vi "Field vs Slow IV.vi"() -> ()   [LabVIEW 2020]
uses:
  <vilib>/Utility/file.llb/Write Delimited Spreadsheet (DBL).vi
panel:
  in  "Tab Control 2":enum32{"Plot 0", "Plot 1", "Plot 2", "Plot 3"}(tab)
  out "I vs Chan 0":cluster{"Y":dbl[], "Y":dbl[]}[](graph)=[{"Y"=[1.5, 1.505, 1.51, 1.515, 1.52, 1.525, 1.53, 1.535, 1.54, 1.545, 1.55, 1.555, 1.56, 1.565, 1.57, 1.575, 1.58, 1.585, 1.59, 1.595, 1.6, 1.605, 1.61, 1.615, 1.62, 1.625, 1.63, 1.635, 1.6400000000000001, 1.645, 1.65, 1.655, 1.66, 1.665, 1.67, 1.675, 1.68, 1.685, 1.69, 1.695, 1.7, 1.705, 1.71, 1.715, 1.72, 1.725, 1.73, 1.735, 1.74, 1.745, 1.75, 1.755, 1.76, 1.7650000000000001, 1.77, 1.775, 1.78, 1.7850000000000001, 1.79, 1.795, 1.8, 1.805, 1.81, 1.815, 1.82, 1.825, 1.83, 1.835, 1.84, 1.845, 1.85, 1.855, 1.8599999999999999, 1.865, 1.87, 1.875, 1.88, 1.885, 1.8900000000000001, 1.895, 1.9, 1.905, 1.9100000000000001, 1.915, 1.92, 1.925, 1.93, 1.935, 1.94, 1.945, 1.95, 1.955, 1.96, 1.965, 1.97, 1.975, 1.98, 1.9849999999999999, 1.99, 1.995, 2.0, 2.005, 2.01, 2.015, 2.02, 2.025, 2.0300000000000002, 2.035, 2.04, 2.045, 2.05, 2.055, 2.06, 2.065, 2.0700000000000003, 2.075, 2.08, 2.085, 2.09, 2.0949999999999998, 2.1, 2.105, 2.11, 2.115, 2.12, 2.125, 2.13, 2.135, 2.14, 2.145, 2.15, 2.1550000000000002, 2.16, 2.165, 2.17, 2.175, 2.18, 2.185, 2.19, 2.1950000000000003, 2.2, 2.205, 2.21, 2.215, 2.2199999999999998, 2.225, 2.23, 2.235, 2.24, 2.245, 2.25, 2.255, 2.26, 2.265, 2.27, 2.275, 2.2800000000000002, 2.285, 2.29, 2.295, 2.3, 2.305, 2.31, 2.315, 2.3200000000000003, 2.325, 2.33, 2.335, 2.34, 2.3449999999999998, 2.35, 2.355, 2.36, 2.365, 2.37, 2.375, 2.38, 2.385, 2.39, 2.395, 2.4, 2.4050000000000002, 2.41, 2.415, 2.42, 2.425, 2.43, 2.435, 2.44, 2.4450000000000003, 2.45, 2.455, 2.46, 2.465, 2.4699999999999998, 2.475, 2.48, 2.485, 2.49, 2.495, 2.5, 2.505, 2.51, 2.515, 2.52, 2.525, 2.5300000000000002, 2.535, 2.54, 2.545, 2.55, 2.5549999999999997, 2.56, 2.565, 2.5700000000000003, 2.575, 2.58, 2.585, 2.59, 2.5949999999999998, 2.6, 2.605, 2.6100000000000003, 2.615, 2.62, 2.625, 2.63, 2.635, 2.64, 2.645, 2.6500000000000004, 2.6550000000000002, 2.66, 2.665, 2.67, 2.675, 2.6799999999999997, 2.685, 2.69, 2.6950000000000003, 2.7, 2.705, 2.71, 2.715, 2.7199999999999998, 2.725, 2.73, 2.7350000000000003, 2.74, 2.745, 2.75, 2.755, 2.76, 2.765, 2.77, 2.7750000000000004, 2.7800000000000002, 2.785, 2.79, 2.795, 2.8, 2.8049999999999997, 2.81, 2.815, 2.8200000000000003, 2.825, 2.83, 2.835, 2.84, 2.8449999999999998, 2.85, 2.855, 2.8600000000000003, 2.865, 2.87, 2.875, 2.88, 2.885, 2.89, 2.895, 2.9000000000000004, 2.9050000000000002, 2.91, 2.915, 2.92, 2.925, 2.9299999999999997, 2.935, 2.94, 2.9450000000000003, 2.95, 2.955, 2.96, 2.965, 2.9699999999999998, 2.975, 2.98, 2.9850000000000003, 2.99, 2.995, 3.0], "Y"=[6.6156494140625e-06, 6.5995361328125006e-06, 6.860595703125e-06, 6.815966796875001e-06, 6.629296875e-06, 6.725463867187501e-06, 6.89208984375e-06, 6.7604248046875e-06, 6.703466796875001e-06, 6.905004882812501e-06, 7.143994140625e-06, 6.781860351562501e-06, 6.9577392578125e-06, 6.8951171875e-06, 7.09951171875e-06, 7.2299072265625e-06, 7.1348144531250006e-06, 7.0348876953125e-06, 7.0186279296875e-06, 6.8879638671874995e-06, 6.9955078125e-06, 7.0866455078125e-06, 7.0669433593750004e-06, 6.9783691406250005e-06, 6.9769287109375e-06, 7.027465820312501e-06, 7.299096679687501e-06, 7.0621826171875e-06, 7.042236328125e-06, 7.05390625e-06, 7.270654296875e-06, 7.450976562500001e-06, 7.242333984375001e-06, 7.214819335937501e-06, 7.214331054687501e-06, 7.0223388671875e-06, 7.086694335937501e-06, 7.0981201171875e-06, 7.3460693359374996e-06, 7.3974609375e-06, 7.264575195312501e-06, 7.3940673828125e-06, 7.2310302734375e-06, 7.469677734375001e-06, 7.527587890625e-06, 7.409790039062501e-06, 7.722314453125e-06, 7.741162109375e-06, 7.538671875e-06, 7.698876953125e-06, 7.79365234375e-06, 7.7605224609375e-06, 7.908154296875001e-06, 7.778735351562502e-06, 7.8468994140625e-06, 7.7814697265625e-06, 7.9154541015625e-06, 7.78876953125e-06, 7.9025390625e-06, 7.7102783203125e-06, 8.0254638671875e-06, 7.81650390625e-06, 7.7733642578125e-06, 7.838427734375e-06, 8.000756835937501e-06, 7.803369140625e-06, 8.1470947265625e-06, 8.122363281250001e-06, 8.015576171875e-06, 8.0428955078125e-06, 7.7995849609375e-06, 8.1434326171875e-06, 8.0010986328125e-06, 7.897656250000001e-06, 7.827612304687501e-06, 7.766748046874999e-06, 7.85146484375e-06, 7.889453125e-06, 7.968872070312499e-06, 8.0005615234375e-06, 8.2376220703125e-06, 8.1786376953125e-06, 8.2513916015625e-06, 8.29208984375e-06, 8.2388671875e-06, 8.19931640625e-06, 8.2802001953125e-06, 8.443017578125001e-06, 8.449755859375e-06, 8.4138916015625e-06, 8.564306640625e-06, 8.4105224609375e-06, 8.2320068359375e-06, 8.366552734375001e-06, 8.518701171875e-06, 8.652294921875002e-06, 8.6939453125e-06, 8.80498046875e-06, 9.227978515625e-06, 9.0858154296875e-06, 9.2788818359375e-06, 9.3503662109375e-06, 9.485009765625e-06, 9.285717773437502e-06, 9.345336914062502e-06, 9.7904296875e-06, 9.7592041015625e-06, 9.6569580078125e-06, 1.01966552734375e-05, 1.03768798828125e-05, 1.013955078125e-05, 1.0394140625000001e-05, 1.0579418945312501e-05, 1.076220703125e-05, 1.073232421875e-05, 1.1024340820312502e-05, 1.1164453125e-05, 1.1322949218750001e-05, 1.1622363281250002e-05, 1.1904931640625e-05, 1.1911572265625002e-05, 1.2339184570312501e-05, 1.2500537109375002e-05, 1.2740844726562501e-05, 1.285322265625e-05, 1.2884936523437502e-05, 1.3046142578125001e-05, 1.3866577148437502e-05, 1.3682031250000003e-05, 1.4437817382812503e-05, 1.4402294921875001e-05, 1.53095947265625e-05, 1.52098876953125e-05, 1.59145263671875e-05, 1.6001611328125e-05, 1.7141601562500003e-05, 1.7263891601562502e-05, 1.71541259765625e-05, 1.8259204101562504e-05, 1.85321044921875e-05, 1.86347412109375e-05, 1.91985107421875e-05, 1.98390380859375e-05, 2.04806396484375e-05, 2.09681640625e-05, 2.2006640625000004e-05, 2.25154296875e-05, 2.27582275390625e-05, 2.3800146484375003e-05, 2.4407739257812502e-05, 2.4760278320312503e-05, 2.57430419921875e-05, 2.6609887695312503e-05, 2.73911376953125e-05, 2.7119091796875e-05, 2.8339111328125e-05, 2.9722607421875003e-05, 3.0245361328125e-05, 3.0236254882812505e-05, 3.1754150390625003e-05, 3.25618408203125e-05, 3.31111572265625e-05, 3.3728198242187504e-05, 3.4521362304687496e-05, 3.520185546875e-05, 3.54622314453125e-05, 3.66463134765625e-05, 3.7109130859375e-05, 3.7485302734375e-05, 3.8547509765625e-05, 3.904365234375e-05, 3.9046875e-05, 3.998369140625e-05, 4.0939404296875e-05, 4.143056640625e-05, 4.179628906250001e-05, 4.2369970703125e-05, 4.26028564453125e-05, 4.3127124023437505e-05, 4.3738183593750005e-05, 4.3873779296875e-05, 4.4547656250000006e-05, 4.45670166015625e-05, 4.54891357421875e-05, 4.6177490234375e-05, 4.6060302734375006e-05, 4.633154296875e-05, 4.6707592773437505e-05, 4.72677978515625e-05, 4.7176904296875e-05, 4.7945458984375005e-05, 4.8335034179687506e-05, 4.86605224609375e-05, 4.8674536132812504e-05, 4.89802978515625e-05, 4.92022705078125e-05, 4.945415039062501e-05, 4.97037353515625e-05, 5.0124487304687504e-05, 5.0323120117187504e-05, 5.0515185546875e-05, 5.0892187499999996e-05, 5.1154541015625e-05, 5.1278369140625e-05, 5.1231542968750003e-05, 5.130100097656251e-05, 5.158137207031251e-05, 5.185832519531251e-05, 5.20868408203125e-05, 5.22366455078125e-05, 5.2339013671875e-05, 5.23698486328125e-05, 5.247021484375e-05, 5.25740966796875e-05, 5.2685058593750004e-05, 5.271892089843751e-05, 5.29219970703125e-05, 5.2985571289062506e-05, 5.3151660156250005e-05, 5.3482714843750004e-05, 5.3514526367187504e-05, 5.373547363281251e-05, 5.39629638671875e-05, 5.41296142578125e-05, 5.41982177734375e-05, 5.42727783203125e-05, 5.43212646484375e-05, 5.462431640625e-05, 5.489465332031251e-05, 5.47357177734375e-05, 5.5075097656250007e-05, 5.5207519531250006e-05, 5.52376708984375e-05, 5.52714599609375e-05, 5.532636718750001e-05, 5.5555004882812503e-05, 5.55648193359375e-05, 5.558767089843751e-05, 5.5666796875000006e-05, 5.5912084960937505e-05, 5.5835253906250005e-05, 5.6077539062500006e-05, 5.6019506835937504e-05, 5.60676513671875e-05, 5.6107861328125e-05, 5.6332250976562506e-05, 5.65072265625e-05, 5.6557568359375e-05, 5.68264404296875e-05, 5.6969409179687504e-05, 5.6886669921875004e-05, 5.7010302734375e-05, 5.707399902343751e-05, 5.70142822265625e-05, 5.7089843750000005e-05, 5.7226318359375e-05, 5.734260253906251e-05, 5.761708984375001e-05, 5.766303710937501e-05, 5.7710791015625e-05, 5.79302734375e-05, 5.7697778320312504e-05, 5.7987426757812505e-05, 5.823701171875e-05, 5.8305810546875005e-05, 5.8348388671874996e-05, 5.84409912109375e-05, 5.8777392578125e-05, 5.8781958007812496e-05, 5.89344482421875e-05, 5.8952099609375e-05, 5.918017578125e-05, 5.92188720703125e-05, 5.954309082031251e-05, 5.977561035156251e-05, 5.9646166992187505e-05, 5.9729345703125005e-05, 5.9951953125e-05, 5.9855004882812506e-05, 5.9770996093749996e-05, 5.99681640625e-05, 6.007705078125e-05, 6.047041015625e-05, 6.06973388671875e-05, 6.0576123046875e-05, 6.0678247070312496e-05, 6.0798999023437506e-05, 6.08008056640625e-05, 6.0889208984375004e-05, 6.09180908203125e-05, 6.10606201171875e-05, 6.12299560546875e-05, 6.111984863281251e-05, 6.12911376953125e-05, 6.16568603515625e-05, 6.173347167968751e-05, 6.18294921875e-05, 6.208735351562501e-05, 6.21252685546875e-05, 6.212973632812499e-05, 6.2308544921875e-05]}]
  out "Name 0":string="DC Voltage V"
  out "I vs Chan 1":cluster{"Y":dbl[], "Y":dbl[]}[](graph)=[{"Y"=[1.5, 1.505, 1.51, 1.515, 1.52, 1.525, 1.53, 1.535, 1.54, 1.545, 1.55, 1.555, 1.56, 1.565, 1.57, 1.575, 1.58, 1.585, 1.59, 1.595, 1.6, 1.605, 1.61, 1.615, 1.62, 1.625, 1.63, 1.635, 1.6400000000000001, 1.645, 1.65, 1.655, 1.66, 1.665, 1.67, 1.675, 1.68, 1.685, 1.69, 1.695, 1.7, 1.705, 1.71, 1.715, 1.72, 1.725, 1.73, 1.735, 1.74, 1.745, 1.75, 1.755, 1.76, 1.7650000000000001, 1.77, 1.775, 1.78, 1.7850000000000001, 1.79, 1.795, 1.8, 1.805, 1.81, 1.815, 1.82, 1.825, 1.83, 1.835, 1.84, 1.845, 1.85, 1.855, 1.8599999999999999, 1.865, 1.87, 1.875, 1.88, 1.885, 1.8900000000000001, 1.895, 1.9, 1.905, 1.9100000000000001, 1.915, 1.92, 1.925, 1.93, 1.935, 1.94, 1.945, 1.95, 1.955, 1.96, 1.965, 1.97, 1.975, 1.98, 1.9849999999999999, 1.99, 1.995, 2.0, 2.005, 2.01, 2.015, 2.02, 2.025, 2.0300000000000002, 2.035, 2.04, 2.045, 2.05, 2.055, 2.06, 2.065, 2.0700000000000003, 2.075, 2.08, 2.085, 2.09, 2.0949999999999998, 2.1, 2.105, 2.11, 2.115, 2.12, 2.125, 2.13, 2.135, 2.14, 2.145, 2.15, 2.1550000000000002, 2.16, 2.165, 2.17, 2.175, 2.18, 2.185, 2.19, 2.1950000000000003, 2.2, 2.205, 2.21, 2.215, 2.2199999999999998, 2.225, 2.23, 2.235, 2.24, 2.245, 2.25, 2.255, 2.26, 2.265, 2.27, 2.275, 2.2800000000000002, 2.285, 2.29, 2.295, 2.3, 2.305, 2.31, 2.315, 2.3200000000000003, 2.325, 2.33, 2.335, 2.34, 2.3449999999999998, 2.35, 2.355, 2.36, 2.365, 2.37, 2.375, 2.38, 2.385, 2.39, 2.395, 2.4, 2.4050000000000002, 2.41, 2.415, 2.42, 2.425, 2.43, 2.435, 2.44, 2.4450000000000003, 2.45, 2.455, 2.46, 2.465, 2.4699999999999998, 2.475, 2.48, 2.485, 2.49, 2.495, 2.5, 2.505, 2.51, 2.515, 2.52, 2.525, 2.5300000000000002, 2.535, 2.54, 2.545, 2.55, 2.5549999999999997, 2.56, 2.565, 2.5700000000000003, 2.575, 2.58, 2.585, 2.59, 2.5949999999999998, 2.6, 2.605, 2.6100000000000003, 2.615, 2.62, 2.625, 2.63, 2.635, 2.64, 2.645, 2.6500000000000004, 2.6550000000000002, 2.66, 2.665, 2.67, 2.675, 2.6799999999999997, 2.685, 2.69, 2.6950000000000003, 2.7, 2.705, 2.71, 2.715, 2.7199999999999998, 2.725, 2.73, 2.7350000000000003, 2.74, 2.745, 2.75, 2.755, 2.76, 2.765, 2.77, 2.7750000000000004, 2.7800000000000002, 2.785, 2.79, 2.795, 2.8, 2.8049999999999997, 2.81, 2.815, 2.8200000000000003, 2.825, 2.83, 2.835, 2.84, 2.8449999999999998, 2.85, 2.855, 2.8600000000000003, 2.865, 2.87, 2.875, 2.88, 2.885, 2.89, 2.895, 2.9000000000000004, 2.9050000000000002, 2.91, 2.915, 2.92, 2.925, 2.9299999999999997, 2.935, 2.94, 2.9450000000000003, 2.95, 2.955, 2.96, 2.965, 2.9699999999999998, 2.975, 2.98, 2.9850000000000003, 2.99, 2.995, 3.0], "Y"=[1.481296142578125, 1.485899658203125, 1.491623779296875, 1.496372802734375, 1.500607421875, 1.506201171875, 1.512212158203125, 1.516510009765625, 1.520935546875, 1.52574560546875, 1.532031982421875, 1.53548974609375, 1.540796630859375, 1.54504443359375, 1.550413818359375, 1.555810546875, 1.5604111328125, 1.56513671875, 1.570776611328125, 1.575748779296875, 1.579657470703125, 1.586687255859375, 1.590750732421875, 1.596195068359375, 1.6001904296875, 1.60581201171875, 1.610980224609375, 1.614694091796875, 1.6195888671875, 1.624559814453125, 1.63003564453125, 1.635827392578125, 1.639400390625, 1.6446259765625, 1.650548828125, 1.654035400390625, 1.659312255859375, 1.664365478515625, 1.6701484375, 1.674442138671875, 1.67888330078125, 1.68497021484375, 1.689583740234375, 1.69438525390625, 1.69949072265625, 1.7033046875, 1.709611328125, 1.7146865234375, 1.719447021484375, 1.724286376953125, 1.728707763671875, 1.733401123046875, 1.738841796875, 1.744190673828125, 1.749333984375, 1.754213623046875, 1.758762451171875, 1.763666015625, 1.768619873046875, 1.773112060546875, 1.778584228515625, 1.78361376953125, 1.788801513671875, 1.793162353515625, 1.79777880859375, 1.801927490234375, 1.808897216796875, 1.8134384765625, 1.817679931640625, 1.823508544921875, 1.82846533203125, 1.833228271484375, 1.838225341796875, 1.843404296875, 1.848100830078125, 1.852965087890625, 1.858184814453125, 1.862722900390625, 1.868026611328125, 1.873251953125, 1.87840966796875, 1.88210595703125, 1.887539794921875, 1.893552001953125, 1.89667529296875, 1.901953369140625, 1.908353515625, 1.9138330078125, 1.917675048828125, 1.923322998046875, 1.92793505859375, 1.934273681640625, 1.9380302734375, 1.942566162109375, 1.948998779296875, 1.9527333984375, 1.957611572265625, 1.963255126953125, 1.9684384765625, 1.972609130859375, 1.97774560546875, 1.9825537109375, 1.987163818359375, 1.99272412109375, 1.996688232421875, 2.00235546875, 2.007000732421875, 2.011778564453125, 2.016716552734375, 2.0221357421875, 2.026481689453125, 2.031533447265625, 2.03667822265625, 2.041638916015625, 2.046490966796875, 2.051802490234375, 2.056508056640625, 2.061195068359375, 2.066268798828125, 2.071982666015625, 2.0766953125, 2.08216748046875, 2.08670263671875, 2.09073828125, 2.096322265625, 2.1008623046875, 2.106653564453125, 2.112296142578125, 2.116163330078125, 2.120879638671875, 2.126167724609375, 2.131207275390625, 2.1357744140625, 2.141315185546875, 2.146663818359375, 2.151198974609375, 2.1564658203125, 2.16050390625, 2.16619970703125, 2.17108447265625, 2.1764951171875, 2.182198486328125, 2.186181640625, 2.191181884765625, 2.19680859375, 2.201070068359375, 2.206341796875, 2.21065283203125, 2.215697021484375, 2.22130908203125, 2.22514111328125, 2.231263671875, 2.235204833984375, 2.24023681640625, 2.246326416015625, 2.250339599609375, 2.25638818359375, 2.25967626953125, 2.26559912109375, 2.270198974609375, 2.275861328125, 2.28002880859375, 2.28554833984375, 2.289510986328125, 2.294212646484375, 2.29975146484375, 2.304468017578125, 2.309668701171875, 2.314978759765625, 2.31974755859375, 2.324486083984375, 2.328228515625, 2.33425634765625, 2.33995361328125, 2.344055419921875, 2.348734619140625, 2.35476513671875, 2.35883203125, 2.36407421875, 2.369318359375, 2.373428955078125, 2.3782236328125, 2.3842890625, 2.389127685546875, 2.394276123046875, 2.398263427734375, 2.40260302734375, 2.408055908203125, 2.413805908203125, 2.418071533203125, 2.42317724609375, 2.42730517578125, 2.432321533203125, 2.4383212890625, 2.443359375, 2.447465576171875, 2.4527998046875, 2.458234130859375, 2.463433349609375, 2.467795654296875, 2.471888427734375, 2.477741455078125, 2.481700927734375, 2.487224365234375, 2.49161474609375, 2.496494873046875, 2.501940185546875, 2.50732861328125, 2.512439697265625, 2.51685888671875, 2.52212939453125, 2.526584716796875, 2.53218310546875, 2.536430908203125, 2.542002197265625, 2.54634326171875, 2.55148583984375, 2.556789794921875, 2.561865478515625, 2.567234619140625, 2.57208447265625, 2.5763681640625, 2.582333251953125, 2.58724560546875, 2.591645751953125, 2.596749755859375, 2.601959228515625, 2.607040283203125, 2.61256787109375, 2.61584228515625, 2.6220859375, 2.626490478515625, 2.630972900390625, 2.636040771484375, 2.641483154296875, 2.6454052734375, 2.65084765625, 2.655864990234375, 2.660786376953125, 2.6665986328125, 2.671231689453125, 2.6759482421875, 2.6809541015625, 2.6863564453125, 2.691091064453125, 2.69605908203125, 2.70098828125, 2.70492822265625, 2.710500732421875, 2.71611083984375, 2.72056298828125, 2.725668212890625, 2.73026123046875, 2.73534423828125, 2.740166748046875, 2.744230224609375, 2.749697509765625, 2.755395751953125, 2.7598564453125, 2.76503271484375, 2.770073486328125, 2.77452294921875, 2.780376708984375, 2.784783203125, 2.790275146484375, 2.79453515625, 2.7993388671875, 2.80516748046875, 2.8095849609375, 2.814790283203125, 2.8197080078125, 2.8248427734375, 2.8291279296875, 2.833797607421875, 2.840931884765625, 2.84431787109375, 2.84849755859375, 2.855468017578125, 2.85949609375, 2.864020751953125, 2.8692666015625, 2.874175537109375, 2.879315673828125, 2.88516943359375, 2.8895234375, 2.89448828125, 2.899353515625, 2.903724853515625, 2.908484619140625, 2.913658203125, 2.919510498046875, 2.9251630859375, 2.92857080078125, 2.934135986328125, 2.939365234375, 2.943295166015625, 2.94798046875, 2.9540498046875, 2.95862841796875, 2.963914794921875, 2.9681767578125]}]
  out "Name 1":string="DC current uA"
  out "I vs Chan 2":cluster{"Y":dbl[], "Y":dbl[]}[](graph)=[{"Y"=[1.5, 1.505, 1.51, 1.515, 1.52, 1.525, 1.53, 1.535, 1.54, 1.545, 1.55, 1.555, 1.56, 1.565, 1.57, 1.575, 1.58, 1.585, 1.59, 1.595, 1.6, 1.605, 1.61, 1.615, 1.62, 1.625, 1.63, 1.635, 1.6400000000000001, 1.645, 1.65, 1.655, 1.66, 1.665, 1.67, 1.675, 1.68, 1.685, 1.69, 1.695, 1.7, 1.705, 1.71, 1.715, 1.72, 1.725, 1.73, 1.735, 1.74, 1.745, 1.75, 1.755, 1.76, 1.7650000000000001, 1.77, 1.775, 1.78, 1.7850000000000001, 1.79, 1.795, 1.8, 1.805, 1.81, 1.815, 1.82, 1.825, 1.83, 1.835, 1.84, 1.845, 1.85, 1.855, 1.8599999999999999, 1.865, 1.87, 1.875, 1.88, 1.885, 1.8900000000000001, 1.895, 1.9, 1.905, 1.9100000000000001, 1.915, 1.92, 1.925, 1.93, 1.935, 1.94, 1.945, 1.95, 1.955, 1.96, 1.965, 1.97, 1.975, 1.98, 1.9849999999999999, 1.99, 1.995, 2.0, 2.005, 2.01, 2.015, 2.02, 2.025, 2.0300000000000002, 2.035, 2.04, 2.045, 2.05, 2.055, 2.06, 2.065, 2.0700000000000003, 2.075, 2.08, 2.085, 2.09, 2.0949999999999998, 2.1, 2.105, 2.11, 2.115, 2.12, 2.125, 2.13, 2.135, 2.14, 2.145, 2.15, 2.1550000000000002, 2.16, 2.165, 2.17, 2.175, 2.18, 2.185, 2.19, 2.1950000000000003, 2.2, 2.205, 2.21, 2.215, 2.2199999999999998, 2.225, 2.23, 2.235, 2.24, 2.245, 2.25, 2.255, 2.26, 2.265, 2.27, 2.275, 2.2800000000000002, 2.285, 2.29, 2.295, 2.3, 2.305, 2.31, 2.315, 2.3200000000000003, 2.325, 2.33, 2.335, 2.34, 2.3449999999999998, 2.35, 2.355, 2.36, 2.365, 2.37, 2.375, 2.38, 2.385, 2.39, 2.395, 2.4, 2.4050000000000002, 2.41, 2.415, 2.42, 2.425, 2.43, 2.435, 2.44, 2.4450000000000003, 2.45, 2.455, 2.46, 2.465, 2.4699999999999998, 2.475, 2.48, 2.485, 2.49, 2.495, 2.5, 2.505, 2.51, 2.515, 2.52, 2.525, 2.5300000000000002, 2.535, 2.54, 2.545, 2.55, 2.5549999999999997, 2.56, 2.565, 2.5700000000000003, 2.575, 2.58, 2.585, 2.59, 2.5949999999999998, 2.6, 2.605, 2.6100000000000003, 2.615, 2.62, 2.625, 2.63, 2.635, 2.64, 2.645, 2.6500000000000004, 2.6550000000000002, 2.66, 2.665, 2.67, 2.675, 2.6799999999999997, 2.685, 2.69, 2.6950000000000003, 2.7, 2.705, 2.71, 2.715, 2.7199999999999998, 2.725, 2.73, 2.7350000000000003, 2.74, 2.745, 2.75, 2.755, 2.76, 2.765, 2.77, 2.7750000000000004, 2.7800000000000002, 2.785, 2.79, 2.795, 2.8, 2.8049999999999997, 2.81, 2.815, 2.8200000000000003, 2.825, 2.83, 2.835, 2.84, 2.8449999999999998, 2.85, 2.855, 2.8600000000000003, 2.865, 2.87, 2.875, 2.88, 2.885, 2.89, 2.895, 2.9000000000000004, 2.9050000000000002, 2.91, 2.915, 2.92, 2.925, 2.9299999999999997, 2.935, 2.94, 2.9450000000000003, 2.95, 2.955, 2.96, 2.965, 2.9699999999999998, 2.975, 2.98, 2.9850000000000003, 2.99, 2.995, 3.0], "Y"=[0.000686767578125, 0.0008046875, 0.00070556640625, 0.000737060546875, 0.0007373046875, 0.00081640625, 0.0007685546875, 0.000751708984375, 0.000693115234375, 0.000705078125, 0.000750732421875, 0.00069140625, 0.000772216796875, 0.000817626953125, 0.000669677734375, 0.00075830078125, 0.00072509765625, 0.000730224609375, 0.000702392578125, 0.000646240234375, 0.0007041015625, 0.000651611328125, 0.000765380859375, 0.0007802734375, 0.000746337890625, 0.000791015625, 0.000671875, 0.000685791015625, 0.000728759765625, 0.0007724609375, 0.00074853515625, 0.00071533203125, 0.000746337890625, 0.000707275390625, 0.0006455078125, 0.000671630859375, 0.000740478515625, 0.00071240234375, 0.000741455078125, 0.000736328125, 0.000663330078125, 0.00077734375, 0.000770263671875, 0.0007431640625, 0.000709716796875, 0.000694580078125, 0.000658203125, 0.000761962890625, 0.000716796875, 0.0007294921875, 0.000708740234375, 0.000719970703125, 0.000759765625, 0.0007119140625, 0.00072509765625, 0.000751220703125, 0.00073046875, 0.00076220703125, 0.000786376953125, 0.000660400390625, 0.00076904296875, 0.0007451171875, 0.000749267578125, 0.000729248046875, 0.000765869140625, 0.00072314453125, 0.00068115234375, 0.0006806640625, 0.00074951171875, 0.000646484375, 0.000708984375, 0.00069287109375, 0.000790283203125, 0.00073828125, 0.00075634765625, 0.0007880859375, 0.00071142578125, 0.00074853515625, 0.000688232421875, 0.00076806640625, 0.000766845703125, 0.000721435546875, 0.00076416015625, 0.000644287109375, 0.0007109375, 0.000718505859375, 0.000741455078125, 0.00070166015625, 0.00070458984375, 0.0007685546875, 0.000790283203125, 0.000731201171875, 0.000719970703125, 0.00076123046875, 0.000741943359375, 0.00072509765625, 0.000703857421875, 0.000728759765625, 0.00071826171875, 0.000761962890625, 0.000738525390625, 0.00075390625, 0.00076953125, 0.000770751953125, 0.000716064453125, 0.000763916015625, 0.000642578125, 0.000780029296875, 0.000813232421875, 0.000796875, 0.0007158203125, 0.0007373046875, 0.000729736328125, 0.00072314453125, 0.000728759765625, 0.000743896484375, 0.0007421875, 0.000664794921875, 0.000705322265625, 0.000717041015625, 0.000751953125, 0.0006923828125, 0.000789794921875, 0.000712890625, 0.000678466796875, 0.00070703125, 0.00078125, 0.000693359375, 0.00076123046875, 0.00076513671875, 0.000746826171875, 0.000696533203125, 0.000743408203125, 0.000717529296875, 0.000701904296875, 0.000748046875, 0.00071044921875, 0.000751708984375, 0.000792724609375, 0.000766357421875, 0.000755859375, 0.00078759765625, 0.000754150390625, 0.00072412109375, 0.000657470703125, 0.0007158203125, 0.000760986328125, 0.00077197265625, 0.000725341796875, 0.000772705078125, 0.0006953125, 0.00079443359375, 0.000690673828125, 0.00071484375, 0.0006767578125, 0.00067626953125, 0.000764892578125, 0.000652099609375, 0.000696533203125, 0.0007265625, 0.000674072265625, 0.000666748046875, 0.0007431640625, 0.00070703125, 0.0007421875, 0.000761962890625, 0.000734619140625, 0.00068212890625, 0.000670166015625, 0.00069287109375, 0.000703125, 0.000656005859375, 0.000713134765625, 0.000716552734375, 0.00072412109375, 0.000741943359375, 0.000707275390625, 0.0007041015625, 0.000737548828125, 0.00070263671875, 0.0007080078125, 0.000760986328125, 0.00073876953125, 0.000724609375, 0.000735595703125, 0.0006669921875, 0.00069287109375, 0.000710693359375, 0.000724365234375, 0.000623779296875, 0.000720458984375, 0.000756591796875, 0.0008076171875, 0.00076123046875, 0.000697509765625, 0.00073974609375, 0.00069873046875, 0.000677001953125, 0.00069970703125, 0.000749755859375, 0.00071435546875, 0.0007197265625, 0.00066015625, 0.000712646484375, 0.000734619140625, 0.00070849609375, 0.00071875, 0.000677490234375, 0.0007197265625, 0.000694091796875, 0.000782958984375, 0.000737060546875, 0.000674560546875, 0.000730712890625, 0.0007265625, 0.000721435546875, 0.000716552734375, 0.00073388671875, 0.00065234375, 0.0007294921875, 0.0007119140625, 0.000756591796875, 0.000716796875, 0.00078857421875, 0.00064599609375, 0.000800537109375, 0.000707275390625, 0.00069189453125, 0.000704345703125, 0.000674560546875, 0.000740234375, 0.0007607421875, 0.000720458984375, 0.000779052734375, 0.0007216796875, 0.0007333984375, 0.000665283203125, 0.000680908203125, 0.000768798828125, 0.00070654296875, 0.000694091796875, 0.00066259765625, 0.000719482421875, 0.000688232421875, 0.000730712890625, 0.0006787109375, 0.000701416015625, 0.00065576171875, 0.000739990234375, 0.00077685546875, 0.00076953125, 0.00064892578125, 0.000725830078125, 0.0006650390625, 0.000781005859375, 0.000702392578125, 0.00065673828125, 0.00071630859375, 0.000720703125, 0.00068115234375, 0.000761474609375, 0.000705078125, 0.00065771484375, 0.000735595703125, 0.000689453125, 0.000717529296875, 0.000713623046875, 0.00070361328125, 0.000772216796875, 0.000658447265625, 0.00068603515625, 0.000721435546875, 0.000724609375, 0.000708740234375, 0.000685546875, 0.00075537109375, 0.00075732421875, 0.000718994140625, 0.0007041015625, 0.0007265625, 0.000692138671875, 0.000771484375, 0.000732177734375, 0.000716064453125, 0.000693603515625, 0.00069091796875, 0.000716552734375, 0.000638427734375, 0.0006689453125, 0.000714111328125, 0.0007451171875, 0.0006875, 0.000751220703125, 0.000694580078125, 0.000660888671875, 0.0006923828125, 0.00068701171875, 0.0006552734375, 0.00069140625, 0.000733154296875, 0.000695068359375]}]
  out "Name 2":string="dV V"
  out "I vs Chan 3":cluster{"Y":dbl[], "Y":dbl[]}[](graph)=[{"Y"=[1.5, 1.505, 1.51, 1.515, 1.52, 1.525, 1.53, 1.535, 1.54, 1.545, 1.55, 1.555, 1.56, 1.565, 1.57, 1.575, 1.58, 1.585, 1.59, 1.595, 1.6, 1.605, 1.61, 1.615, 1.62, 1.625, 1.63, 1.635, 1.6400000000000001, 1.645, 1.65, 1.655, 1.66, 1.665, 1.67, 1.675, 1.68, 1.685, 1.69, 1.695, 1.7, 1.705, 1.71, 1.715, 1.72, 1.725, 1.73, 1.735, 1.74, 1.745, 1.75, 1.755, 1.76, 1.7650000000000001, 1.77, 1.775, 1.78, 1.7850000000000001, 1.79, 1.795, 1.8, 1.805, 1.81, 1.815, 1.82, 1.825, 1.83, 1.835, 1.84, 1.845, 1.85, 1.855, 1.8599999999999999, 1.865, 1.87, 1.875, 1.88, 1.885, 1.8900000000000001, 1.895, 1.9, 1.905, 1.9100000000000001, 1.915, 1.92, 1.925, 1.93, 1.935, 1.94, 1.945, 1.95, 1.955, 1.96, 1.965, 1.97, 1.975, 1.98, 1.9849999999999999, 1.99, 1.995, 2.0, 2.005, 2.01, 2.015, 2.02, 2.025, 2.0300000000000002, 2.035, 2.04, 2.045, 2.05, 2.055, 2.06, 2.065, 2.0700000000000003, 2.075, 2.08, 2.085, 2.09, 2.0949999999999998, 2.1, 2.105, 2.11, 2.115, 2.12, 2.125, 2.13, 2.135, 2.14, 2.145, 2.15, 2.1550000000000002, 2.16, 2.165, 2.17, 2.175, 2.18, 2.185, 2.19, 2.1950000000000003, 2.2, 2.205, 2.21, 2.215, 2.2199999999999998, 2.225, 2.23, 2.235, 2.24, 2.245, 2.25, 2.255, 2.26, 2.265, 2.27, 2.275, 2.2800000000000002, 2.285, 2.29, 2.295, 2.3, 2.305, 2.31, 2.315, 2.3200000000000003, 2.325, 2.33, 2.335, 2.34, 2.3449999999999998, 2.35, 2.355, 2.36, 2.365, 2.37, 2.375, 2.38, 2.385, 2.39, 2.395, 2.4, 2.4050000000000002, 2.41, 2.415, 2.42, 2.425, 2.43, 2.435, 2.44, 2.4450000000000003, 2.45, 2.455, 2.46, 2.465, 2.4699999999999998, 2.475, 2.48, 2.485, 2.49, 2.495, 2.5, 2.505, 2.51, 2.515, 2.52, 2.525, 2.5300000000000002, 2.535, 2.54, 2.545, 2.55, 2.5549999999999997, 2.56, 2.565, 2.5700000000000003, 2.575, 2.58, 2.585, 2.59, 2.5949999999999998, 2.6, 2.605, 2.6100000000000003, 2.615, 2.62, 2.625, 2.63, 2.635, 2.64, 2.645, 2.6500000000000004, 2.6550000000000002, 2.66, 2.665, 2.67, 2.675, 2.6799999999999997, 2.685, 2.69, 2.6950000000000003, 2.7, 2.705, 2.71, 2.715, 2.7199999999999998, 2.725, 2.73, 2.7350000000000003, 2.74, 2.745, 2.75, 2.755, 2.76, 2.765, 2.77, 2.7750000000000004, 2.7800000000000002, 2.785, 2.79, 2.795, 2.8, 2.8049999999999997, 2.81, 2.815, 2.8200000000000003, 2.825, 2.83, 2.835, 2.84, 2.8449999999999998, 2.85, 2.855, 2.8600000000000003, 2.865, 2.87, 2.875, 2.88, 2.885, 2.89, 2.895, 2.9000000000000004, 2.9050000000000002, 2.91, 2.915, 2.92, 2.925, 2.9299999999999997, 2.935, 2.94, 2.9450000000000003, 2.95, 2.955, 2.96, 2.965, 2.9699999999999998, 2.975, 2.98, 2.9850000000000003, 2.99, 2.995, 3.0], "Y"=[0.00172412109375, 0.001721435546875, 0.00168603515625, 0.00166357421875, 0.00168310546875, 0.001632080078125, 0.001675048828125, 0.0017109375, 0.0016943359375, 0.001686767578125, 0.00173095703125, 0.001705322265625, 0.001647705078125, 0.001672607421875, 0.0016767578125, 0.0016572265625, 0.00168896484375, 0.0016826171875, 0.001687255859375, 0.001647705078125, 0.00169775390625, 0.00166357421875, 0.00173388671875, 0.0017080078125, 0.001659912109375, 0.00169140625, 0.0016962890625, 0.001697509765625, 0.001662841796875, 0.00162939453125, 0.0017177734375, 0.001651611328125, 0.00163818359375, 0.001712646484375, 0.001668701171875, 0.00170361328125, 0.001758056640625, 0.001680908203125, 0.001697265625, 0.001639404296875, 0.001704833984375, 0.001695556640625, 0.001661376953125, 0.001728515625, 0.001750244140625, 0.001653564453125, 0.001721435546875, 0.0017109375, 0.001679443359375, 0.001676513671875, 0.0016865234375, 0.001657958984375, 0.001687255859375, 0.001693115234375, 0.00168798828125, 0.00168359375, 0.00169287109375, 0.001712158203125, 0.00172216796875, 0.001672119140625, 0.001680419921875, 0.001711181640625, 0.001709716796875, 0.00168896484375, 0.001654052734375, 0.001686279296875, 0.00166357421875, 0.0016826171875, 0.001654296875, 0.001711181640625, 0.001636474609375, 0.001697509765625, 0.00170361328125, 0.001681884765625, 0.001663818359375, 0.00164111328125, 0.001682373046875, 0.00169189453125, 0.001673095703125, 0.001668701171875, 0.001681884765625, 0.00164404296875, 0.001693115234375, 0.00165283203125, 0.00164501953125, 0.00166064453125, 0.001638427734375, 0.0016728515625, 0.00165087890625, 0.001656005859375, 0.001697265625, 0.001666259765625, 0.001629638671875, 0.001615966796875, 0.00169580078125, 0.00165869140625, 0.001694580078125, 0.0016787109375, 0.001703125, 0.00165966796875, 0.00172705078125, 0.001748779296875, 0.00166015625, 0.00170166015625, 0.0016787109375, 0.001710693359375, 0.00170654296875, 0.001665771484375, 0.00166455078125, 0.001759765625, 0.00169921875, 0.00166162109375, 0.00172705078125, 0.001671875, 0.001734619140625, 0.001705322265625, 0.001665283203125, 0.001691162109375, 0.001689208984375, 0.001666748046875, 0.001759033203125, 0.001675048828125, 0.001667236328125, 0.0016767578125, 0.001724853515625, 0.00165673828125, 0.001669189453125, 0.001679931640625, 0.001667724609375, 0.00168603515625, 0.001764404296875, 0.00171826171875, 0.001695068359375, 0.00172802734375, 0.00165771484375, 0.001701904296875, 0.001660888671875, 0.001697265625, 0.00170556640625, 0.00173388671875, 0.00172314453125, 0.001640380859375, 0.001629638671875, 0.00165966796875, 0.00167529296875, 0.001738525390625, 0.001657958984375, 0.001710693359375, 0.00167724609375, 0.001677490234375, 0.00166943359375, 0.001637939453125, 0.001658935546875, 0.001703125, 0.001694091796875, 0.001676025390625, 0.00168310546875, 0.00167578125, 0.001646240234375, 0.001751953125, 0.0016689453125, 0.00170361328125, 0.001697021484375, 0.001707763671875, 0.001684326171875, 0.001719970703125, 0.001631591796875, 0.001638427734375, 0.001682861328125, 0.00175537109375, 0.0016767578125, 0.0017099609375, 0.001689697265625, 0.00172119140625, 0.001761962890625, 0.001656982421875, 0.001688232421875, 0.001677978515625, 0.00167919921875, 0.0016611328125, 0.001636962890625, 0.001694580078125, 0.001733154296875, 0.001700927734375, 0.001701171875, 0.001706298828125, 0.00170263671875, 0.001689208984375, 0.001663818359375, 0.001662353515625, 0.0017177734375, 0.00167041015625, 0.001654052734375, 0.001680419921875, 0.0017236328125, 0.0016943359375, 0.0016875, 0.001731201171875, 0.001698974609375, 0.001718505859375, 0.001677001953125, 0.001695556640625, 0.001710693359375, 0.001684814453125, 0.001716064453125, 0.001660400390625, 0.001641845703125, 0.001656982421875, 0.001673095703125, 0.001685302734375, 0.00160498046875, 0.00165380859375, 0.0017490234375, 0.001673583984375, 0.001743408203125, 0.00170361328125, 0.001679931640625, 0.001680419921875, 0.001702392578125, 0.001679931640625, 0.001658935546875, 0.001725341796875, 0.001708251953125, 0.001735107421875, 0.001676025390625, 0.001728515625, 0.00171533203125, 0.0016328125, 0.001673583984375, 0.001707275390625, 0.001645751953125, 0.001700927734375, 0.001675537109375, 0.001673583984375, 0.001682861328125, 0.001618408203125, 0.001680908203125, 0.0016806640625, 0.00168115234375, 0.00167041015625, 0.00169873046875, 0.00166552734375, 0.00168701171875, 0.0017099609375, 0.00169921875, 0.001651123046875, 0.001683837890625, 0.0016748046875, 0.001654541015625, 0.001683349609375, 0.001668212890625, 0.00162548828125, 0.00167333984375, 0.0016435546875, 0.0016689453125, 0.0017265625, 0.001734619140625, 0.001675537109375, 0.0016943359375, 0.001693359375, 0.001719970703125, 0.001652099609375, 0.001674560546875, 0.001696533203125, 0.001704345703125, 0.001668212890625, 0.001690185546875, 0.001684326171875, 0.001725830078125, 0.0017099609375, 0.001635009765625, 0.00161328125, 0.001689208984375, 0.00168017578125, 0.001648681640625, 0.0016796875, 0.00165576171875, 0.0016513671875, 0.001722412109375, 0.00173046875, 0.001647216796875, 0.00166748046875, 0.00167236328125, 0.001693603515625, 0.001658447265625, 0.001661865234375, 0.00169970703125, 0.00171142578125, 0.001665771484375, 0.001665771484375, 0.001686279296875, 0.00163916015625, 0.00164208984375, 0.001709228515625, 0.0016494140625, 0.001640869140625, 0.001671142578125, 0.001713134765625, 0.001692626953125, 0.00167919921875, 0.0016806640625]}]
  out "Name 3":string="dI uA"
  in  "Tab Control":T1(tab)=enum."Field"
  in  "cRIO IP":string="//172.22.11.2"
  in  "Reading Average times":i32=1000
  in  "Current Start uA":dbl=1.5
  in  "Current Range uA":dbl=1.5
  in  "Current Step uA":dbl=0.005
  in  "Current output Scale factor":dbl=1.0
  in  "Ramp type":string(combo)="Range"
  in  "Ramp up first T":bool=TRUE
  in  "AO Channel":string(combo)="AO0"
  in  "Delay Time s":dbl=0.15 caption="Delay Time (s)"
  in  "Channel name 0":string(combo)="DC Voltage V"
  in  "Scale factor0":dbl=0.0001
  in  "Chan 1":bool=TRUE
  in  "Channel name 1":string(combo)="DC current uA"
  in  "Scale factor1":dbl=1.0
  in  "Chan 2":bool
  in  "Channel name 2":string(combo)="dV V"
  in  "Scale factor2":dbl=1.0
  in  "Chan 3":bool
  in  "Channel name 3":string(combo)="dI uA"
  in  "Scale factor3":dbl=1.0
  in  "Contour plot folder":path=path "C:/Users/gyue/Desktop/Data folder 20210720"
  in  "Book name":string="book723"
  in  "Current VI path":path=path "C:/Users/gyue/Box/Guang Yue uiuc research box folder/Labview/cRIO related/Field vs Slow IV.vi"
  out "Current Field mT":dbl=0.30000000000000004
  in  "stop":bool
  in  "Ramp up first T 2":bool=TRUE
  in  "Ramp type 2":string(combo)="Range"
  in  "Field Origin mT":dbl=0.2 format="%#_13g"
  in  "Field step mT":dbl=0.0005 format="%#_13g"
  in  "Field Radius mT":dbl=0.1 format="%#_13g"
  in  "Field Rate mT per sec":dbl=0.1 format="%#_13g"
  in  "Magnet Device Select":string(combo)="NI DAQ Controlled V to I source"
  out "error out":errorcluster
  # "Voltage x factor=uA"
  # "Voltage x factor=actual"
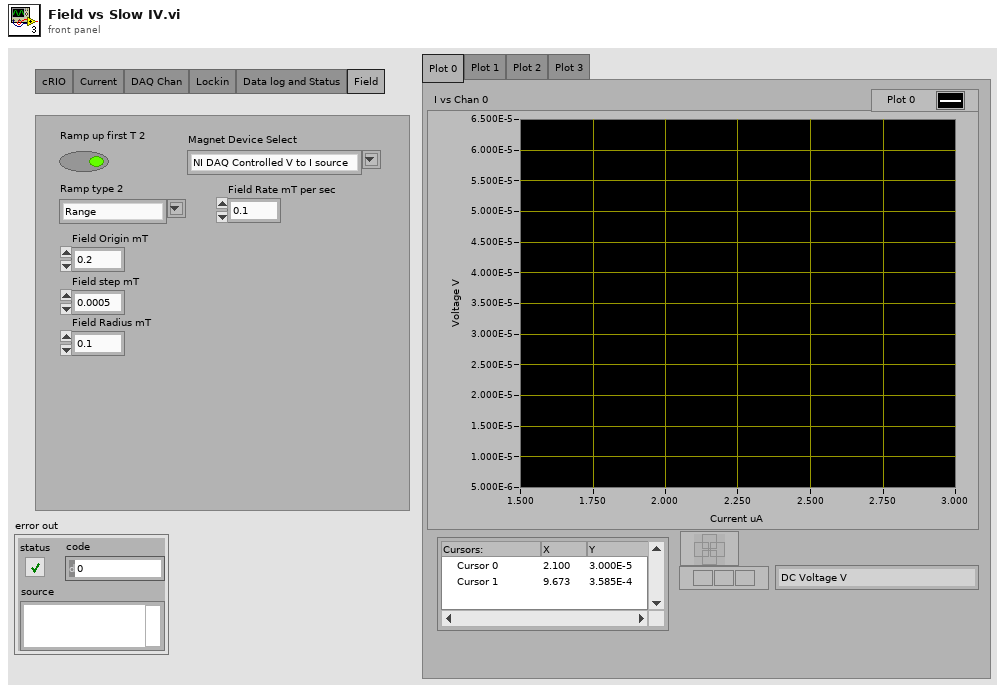
[diagram p1: front panel]
types:
  T1 = enum32{"cRIO", "Current", "DAQ Chan", "Lockin", "Data log and Status", "Field"}
  T2 = cluster{"AI0":dbl, "AI1":dbl, "AI2":dbl, "AI3":dbl}
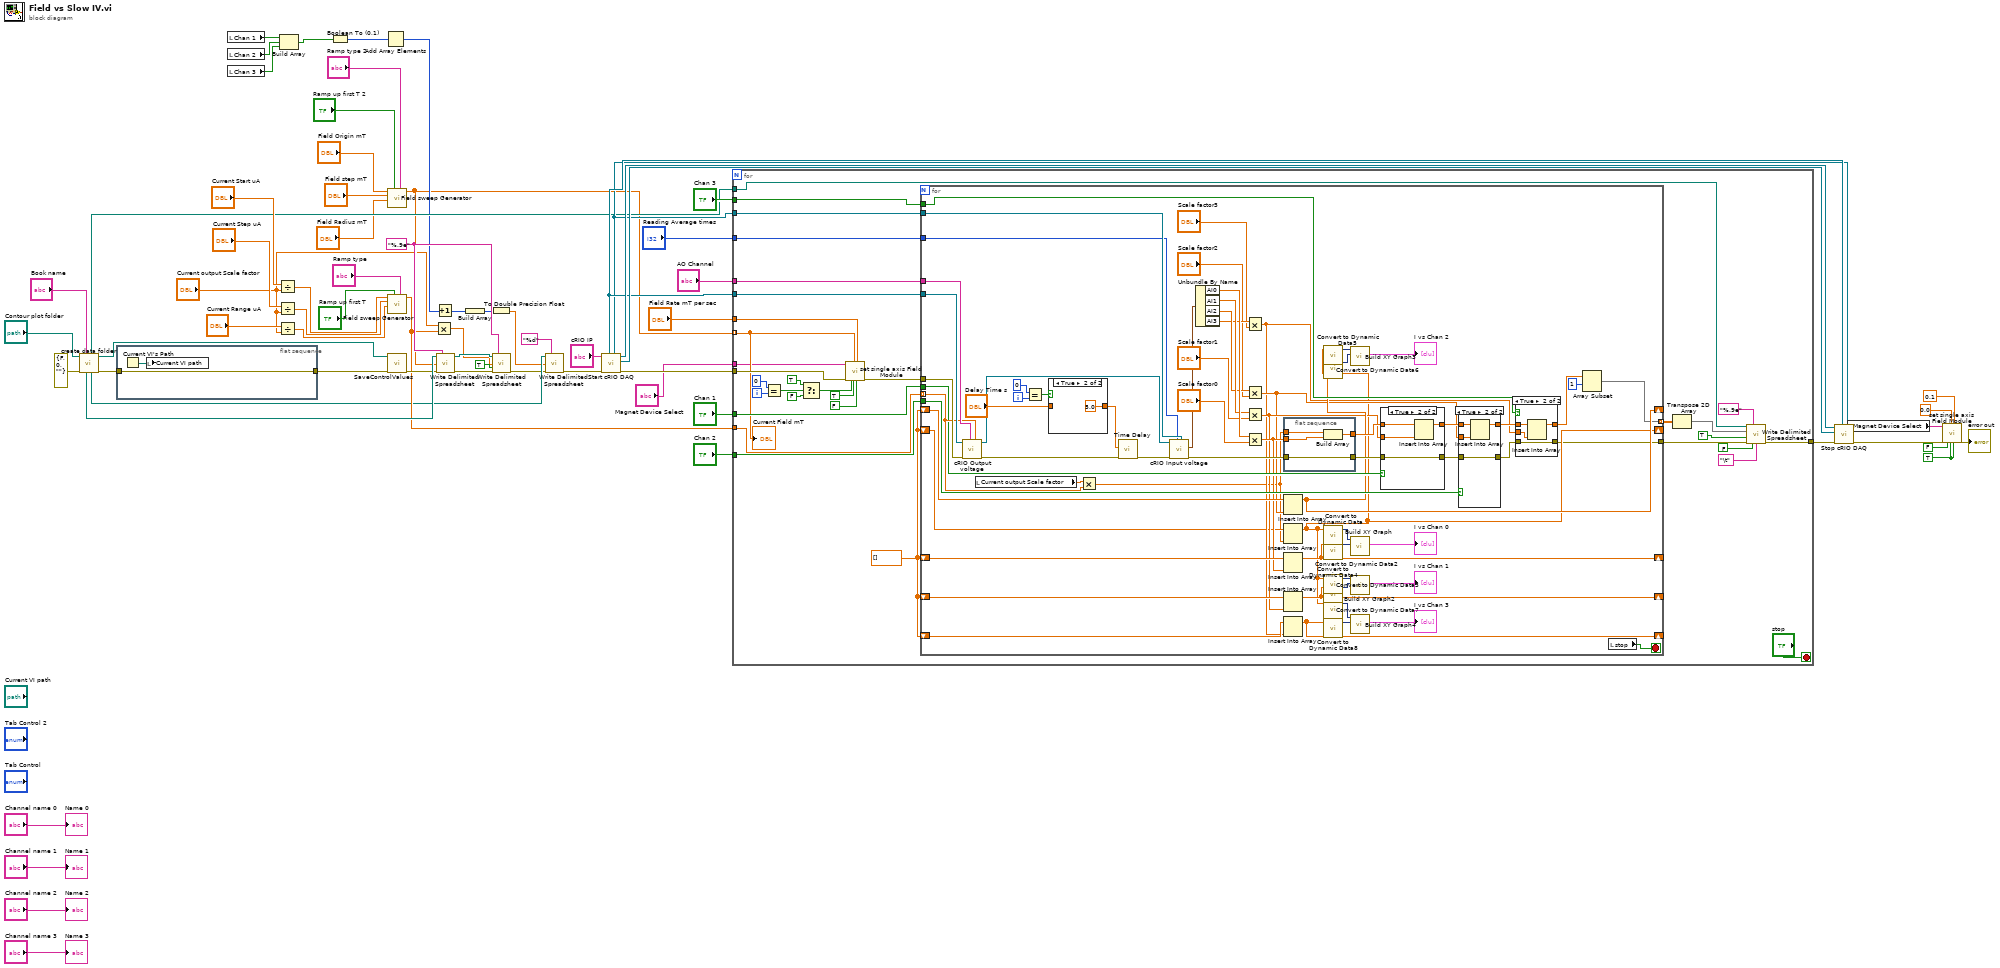
[diagram p0: block diagram]
diagram:
  w2 = TRUE ("final")
  w30 = "%.9e" ("format (%.3f)")
  n1 = call "create data folder.vi"("Name"="Book name", "error in"=errorcluster {"status"=FALSE, "code"=0, "source"=""}, "Contour plot folder"="Contour plot folder") -> ("error out"=w39:errorcluster, "xml path"=w41:path, "book par"=w24:path, "IV path"=w40:path, "Field path"=w37:path)  [unwired: 4 in]
  n2 = flat-sequence {
    tunnel: w39 -> [w69]
    tunnel: [w69] -> w38
    frame #0 {
      n3 = Current VI's Path() -> (path=w70:path)
      n4 = local write "Current VI path"(w70) -> ()
    }
  }
  n5 = local read "Chan 1"() -> (w22:bool)
  n6 = local read "Chan 2"() -> (w21:bool)
  n7 = local read "Chan 3"() -> (w20:bool)
  n8 = Divide(x="Current Start uA", y="Current output Scale factor") -> (x/y=w60:dbl)
  n9 = Divide(x="Current Step uA", y="Current output Scale factor") -> (x/y=w59:dbl)
  n10 = Divide(x="Current Range uA", y="Current output Scale factor") -> (x/y=w58:dbl)
  n11 = Build Array(w22, w21, w20) -> (w19:bool[])
  n12 = Boolean To (0,1)(Boolean=w19) -> (0, 1=w18:i16[])
  n13 = Add Array Elements(numeric array=w18) -> (sum=w17:i16)
  n14 = call "Field sweep Generator.vi"("Ramp type"="Ramp type 2", "Ramp up first T"="Ramp up first T 2", "Field Radius"="Field Radius mT", "Field step"="Field step mT", "Field Origin"="Field Origin mT") -> ("output array"=w12:dbl[])  [unwired: 6 in]
  n15 = call "Field sweep Generator.vi"("Ramp type"="Ramp type", "Ramp up first T"="Ramp up first T", "Field Radius"=w58, "Field step"=w59, "Field Origin"=w60) -> ("output array"=w28:dbl[])  [unwired: 6 in]
  n16 = call "SaveControlValues.vi"("XML File Path"=w41, "error in (no error)"=w38) -> ("error out"=w36:errorcluster)  [unwired: 8 in]
  n17 = Multiply(x="Current output Scale factor", y=w28) -> (x*y=w5:dbl[])
  n18 = Increment(x=w17) -> (x+1=w16:i16)
  n19 = call-poly <vilib>:"Write Delimited Spreadsheet.vi"("file path (dialog if empty)"=w37, "format (%.3f)"=w30, "1D data"=w12, "error in (no error)"=w36) -> ("new file path (Not A Path if cancelled)"=w29:path, "error out"=w26:errorcluster)  [unwired: 10 in]
  n20 = Build Array(w16) -> (w15:i16[])
  n21 = To Double Precision Float(number=w15) -> (double precision float=w14:dbl[])
  n22 = call-poly <vilib>:"Write Delimited Spreadsheet.vi"("file path (dialog if empty)"=w29, "format (%.3f)"=w30, "1D data"=w5, "append to file? (new file:F)"=TRUE, "error in (no error)"=w26) -> ("error out"=w23:errorcluster)  [unwired: 9 in, 1 out]
  n23 = call-poly <vilib>:"Write Delimited Spreadsheet.vi"("file path (dialog if empty)"=w24, "format (%.3f)"="%d", "1D data"=w14, "error in (no error)"=w23) -> ("error out"=w13:errorcluster)  [unwired: 10 in, 1 out]
  n24 = call "Start cRIO DAQ.vi"("error in (no error)"=w13, "cRIO IP"="cRIO IP") -> ("error out"=w57:errorcluster, "vi reference"=w67:refnum<vi>, "application reference"=w68:refnum<vi>, "DAQ_AI_Reader endpoint"=w54:refnum<k21>, "DAQ_CMD_Writer endpoint"=w55:refnum<k21>)  [unwired: 5 in]
  n25 = for {
    tunnel: "AO Channel" -> [w102]
    tunnel: w28 -> [w101]
    tunnel: w55 -> [w100]
    tunnel: w54 -> [w99]
    tunnel: "Chan 1" -> [w98]
    tunnel: "Chan 2" -> [w97]
    tunnel: "Chan 3" -> [w96]
    tunnel: "Reading Average times" -> [w94]
    tunnel: w40 -> [w88]
    tunnel: w12 -> [w90] mode=indexing
    tunnel: w57 -> [w92]
    tunnel: [w82] -> w50
    tunnel: "Field Rate mT per sec" -> [w91]
    tunnel: "Magnet Device Select" -> [w71]
    i -> [w77]
    stop <- "stop" stop-if-true
    w95 = dbl[] []
    n26 = Equal?(x=0, y=w77) -> (x = y?=w75:bool)
    n27 = Select(t=TRUE ("Init"), s=w75, f=FALSE) -> (s? t:f=w72:bool)
    n28 = call "set single axis Field Module.vi"("Magnet Device Select"=w71, "error in (no error)"=w92, "Init"=w72, "Field Target mT"=w90, "Exec"=TRUE, "Field Rate mT per sec"=w91, "final"=FALSE) -> ("error out"=w89:errorcluster)  [unwired: 12 in]
    n29 = for {
      tunnel: w89 -> [w168]
      tunnel: w100 -> [w167]
      tunnel: w102 -> [w166]
      tunnel: w101 -> [w156] mode=indexing
      tunnel: w99 -> [w164]
      tunnel: w98 -> [w147]
      tunnel: w97 -> [w146]
      tunnel: w96 -> [w145]
      shift-right: [w124] -> _
      shift-left: w95 -> [w128]
      shift-right: [w123] -> _
      shift-left: w95 -> [w127]
      shift-right: [w122] -> _
      shift-left: w95 -> [w126]
      shift-right: [w121] -> _
      shift-left: w95 -> [w125]
      shift-right: [w114] -> _
      shift-left: w95 -> [w116]
      tunnel: w94 -> [w113]
      tunnel: [w109] -> w81 mode=indexing
      tunnel: [w112] -> w85
      i -> [w107]
      stop <- w103 stop-if-true
      n30 = call "cRIO Output voltage.vi"("Voltage"=w156, "AO Channel"=w166, "error in (no error)"=w168, "DAQ_CMD_Writer endpoint"=w167) -> ("error out"=w160:errorcluster, "DAQ_CMD_Writer endpoint out"=w165:refnum<k21>)  [unwired: 6 in]
      n31 = local read "Current output Scale factor"() -> (w157:dbl)
      n32 = Equal?(x=0, y=w107) -> (x = y?=w106:bool)
      n33 = case shown="True" w106 {
        tunnel: "Delay Time s" -> [w169 _]
        tunnel: [w169 5.0 ("Delay Time s")] -> w104
        frame False {
        }
        frame True {
        }
      }
      n34 = Multiply(x=w157, y=w156) -> (x*y=w115:dbl)
      n35 = call "Time Delay"("error in (no error)"=w160, "Delay Time (s)"=w104) -> ("error out"=w159:errorcluster)  [unwired: 9 in]
      n36 = call "cRIO Input voltage.vi"("DAQ_AI_Reader endpoint"=w164, "Average"=w113, "error in (no error)"=w159, "DAQ_CMD_Writer endpoint"=w165) -> ("error out"=w142:errorcluster, "output cluster"=w158:T2)  [unwired: 5 in, 1 out]
      n37 = Unbundle By Name(w158) -> ("AI0"=w155:dbl, "AI1"=w154:dbl, "AI2"=w153:dbl, "AI3"=w152:dbl)
      n38 = Multiply(x=w152, y="Scale factor3") -> (x*y=w117:dbl)
      n39 = Multiply(x=w153, y="Scale factor2") -> (x*y=w118:dbl)
      n40 = Multiply(x=w154, y="Scale factor1") -> (x*y=w119:dbl)
      n41 = Multiply(x=w155, y="Scale factor0") -> (x*y=w120:dbl)
      n42 = flat-sequence {
        tunnel: w142 -> [w174]
        tunnel: [w174] -> w141
        tunnel: w120 -> [w172]
        tunnel: [w173] -> w140
        tunnel: w115 -> [w171]
        frame #0 {
          n43 = Build Array(w171, w172) -> (w173:dbl[])
        }
      }
      n44 = Insert Into Array(array=w126, new element=w118) -> (w122:dbl[])  [unwired: 1 in]
      n45 = Insert Into Array(array=w116, new element=w115) -> (w114:dbl[])  [unwired: 1 in]
      n46 = Insert Into Array(array=w128, new element=w120) -> (w124:dbl[])  [unwired: 1 in]
      n47 = Insert Into Array(array=w127, new element=w119) -> (w123:dbl[])  [unwired: 1 in]
      n48 = Insert Into Array(array=w125, new element=w117) -> (w121:dbl[])  [unwired: 1 in]
      n49 = call "Convert to Dynamic Data5"("Array"=w114) -> ("Dynamic Data Type"=w133:dynamicdata)  [unwired: 3 in]
      n50 = call "Convert to Dynamic Data6"("Array"=w122) -> ("Dynamic Data Type"=w134:dynamicdata)  [unwired: 3 in]
      n51 = call "Convert to Dynamic Data"("Array"=w114) -> ("Dynamic Data Type"=w162:dynamicdata)  [unwired: 3 in]
      n52 = call "Convert to Dynamic Data2"("Array"=w124) -> ("Dynamic Data Type"=w163:dynamicdata)  [unwired: 3 in]
      n53 = call "Convert to Dynamic Data3"("Array"=w114) -> ("Dynamic Data Type"=w136:dynamicdata)  [unwired: 3 in]
      n54 = call "Convert to Dynamic Data4"("Array"=w123) -> ("Dynamic Data Type"=w137:dynamicdata)  [unwired: 3 in]
      n55 = call "Convert to Dynamic Data7"("Array"=w114) -> ("Dynamic Data Type"=w130:dynamicdata)  [unwired: 3 in]
      n56 = call "Convert to Dynamic Data8"("Array"=w121) -> ("Dynamic Data Type"=w131:dynamicdata)  [unwired: 3 in]
      n57 = call "Build XY Graph3"("Y Input"=w134, "X Input"=w133) -> ("XY Graph"=→"I vs Chan 2":cluster{"X":dbl[], "Y":dbl[]}[])  [unwired: 8 in, 1 out]
      n58 = call "Build XY Graph"("Y Input"=w163, "X Input"=w162) -> ("XY Graph"=→"I vs Chan 0":cluster{"X":dbl[], "Y":dbl[]}[])  [unwired: 8 in, 1 out]
      n59 = call "Build XY Graph2"("Y Input"=w137, "X Input"=w136) -> ("XY Graph"=→"I vs Chan 1":cluster{"X":dbl[], "Y":dbl[]}[])  [unwired: 8 in, 1 out]
      n60 = call "Build XY Graph4"("Y Input"=w131, "X Input"=w130) -> ("XY Graph"=→"I vs Chan 3":cluster{"X":dbl[], "Y":dbl[]}[])  [unwired: 8 in, 1 out]
      n61 = case shown="True" w147 {
        tunnel: w141 -> [w187 w192]
        tunnel: [w187 w192] -> w144
        tunnel: w140 -> [w188 w191]
        tunnel: w119 -> [_ w190]
        tunnel: [w188 w189] -> w139
        frame False {
        }
        frame True {
          n62 = Insert Into Array(array=w191, new element=w190) -> (w189:dbl[])  [unwired: 1 in]
        }
      }
      n63 = case shown="True" w146 {
        tunnel: w144 -> [w181 w186]
        tunnel: [w181 w186] -> w143
        tunnel: w139 -> [w182 w185]
        tunnel: w118 -> [_ w184]
        tunnel: [w182 w183] -> w138
        frame False {
        }
        frame True {
          n64 = Insert Into Array(array=w185, new element=w184) -> (w183:dbl[])  [unwired: 1 in]
        }
      }
      n65 = case shown="True" w145 {
        tunnel: w143 -> [w175 w177]
        tunnel: w138 -> [w176 w180]
        tunnel: w117 -> [_ w179]
        tunnel: [w176 w178] -> w111
        tunnel: [w175 w177] -> w112
        frame False {
        }
        frame True {
          n66 = Insert Into Array(array=w180, new element=w179) -> (w178:dbl[])  [unwired: 1 in]
        }
      }
      n67 = Array Subset(array=w111, index=1) -> (w109:dbl[])  [unwired: 1 in]
      n68 = local read "stop"() -> (w103:bool)
    }
    n69 = Transpose 2D Array(2D array=w81) -> (transposed array=w80:dbl[][])
    n70 = call-poly <vilib>:"Write Delimited Spreadsheet.vi"("file path (dialog if empty)"=w88, "format (%.3f)"="%.9e", "2D data"=w80, "append to file? (new file:F)"=TRUE, "error in (no error)"=w85, "transpose? (no:F)"=FALSE, "delimiter (\\t)"="\t" ("delimiter (\\t)")) -> ("error out"=w82:errorcluster)  [unwired: 7 in, 1 out]
    "Current Field mT" <- w90
  }
  n71 = call "Stop cRIO DAQ.vi"("DAQ_AI_Reader endpoint"=w54, "DAQ_CMD_Writer endpoint"=w55, "error in (no error)"=w50, "VI reference"=w67, "application reference"=w68) -> ("error out"=w10:errorcluster)  [unwired: 6 in]
  n72 = local read "Magnet Device Select"() -> (w8:string)
  n73 = call "set single axis Field Module.vi"("Magnet Device Select"=w8, "error in (no error)"=w10, "Init"=FALSE, "Field Target mT"=0.0, "Exec"=w2, "Field Rate mT per sec"=0.1, "final"=w2) -> ("error out"=→"error out":errorcluster)  [unwired: 12 in]
  "Name 0" <- "Channel name 0"
  "Name 1" <- "Channel name 1"
  "Name 2" <- "Channel name 2"
  "Name 3" <- "Channel name 3"
